vi "SRV_Build iw Command Data.vi"(0 "Motor Control Command":T1={"I2C Address"=0, "Register"=0, "Value"=0, "Active"=TRUE} {"Value" format="%02x"; "Register" format="%02x"; "I2C Address" format="%02x"}) -> (6 "Command Data String":string, 8 "iw Command Data Field":u8[](array[numeric]) format="%02x", 10 "Active":bool)   [LabVIEW 2009]
doc: "<B>iwabc</B>\nI2C register write ('abc' parameters sent as 8-bit binary)\na is device id, b is register, c is value written to register\n\n\nAuthor: Mike Schultz (LogicPD, Inc)"
uses:
  Motors Config/SRV_Motor Control Command Config.ctl
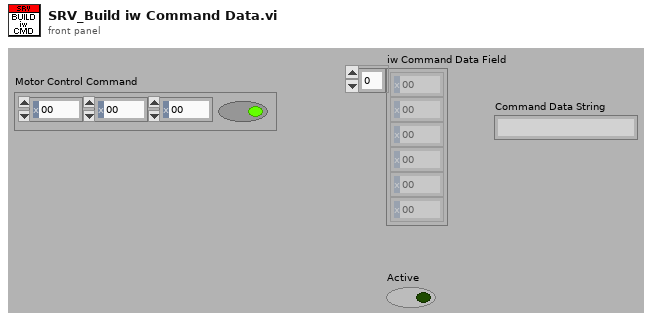
[diagram p1: front panel]
types:
  T1 = typedef "SRV_Motor Control Command Config.ctl" = cluster{"I2C Address":u8, "Register":u8, "Value":u8, "Active":bool}
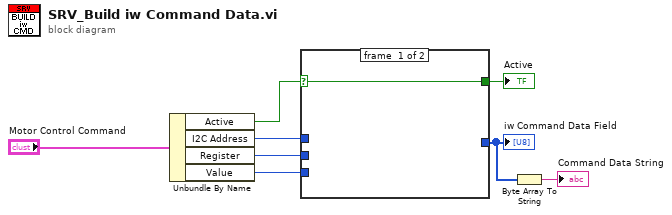
[diagram p0: block diagram]
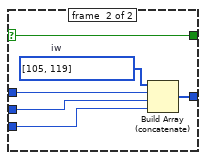
[diagram p2: hidden frame]
diagram:
  n1 = Unbundle By Name("Motor Control Command") -> ("Active"=w7:bool, "I2C Address"=w6:u8, "Register"=w5:u8, "Value"=w4:u8)
  n2 = case shown="True" w7 {
    selector: w7 -> [w9 w11]
    tunnel: w6 -> [_ w15]
    tunnel: w5 -> [_ w14]
    tunnel: w4 -> [_ w13]
    tunnel: [_ w12] -> w2
    tunnel: [w9 w11] -> w3
    frame #0 {
    }
    frame #1 {
      w10 = u8[] [105, 119]  # iw
      n3 = Build Array (concatenate)(w10, w15, w14, w13) -> (w12:u8[])
    }
  }
  "iw Command Data Field" <- w2
  "Active" <- w3
  n4 = Byte Array To String(unsigned byte array=w2) -> (string=→"Command Data String":string)
